vi "Wavelet Transform Daubechies4.vi"(0 "X":dbl[](array[numeric])) -> (1 "Wavelet Daubechies4 {X}":dbl[](array[numeric]), 2 "error":i32)   [LabVIEW 2010, in "NI_Gmath.lvlib"]
doc: "Computes the wavelet transform based on the Daubechies4 function of the input sequence <B>X</B>."
uses:
  NI_Gmath.lvlib
  Real Dot Product.vi
  NI_AALBase.lvlib
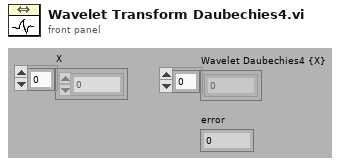
[diagram p1: front panel]
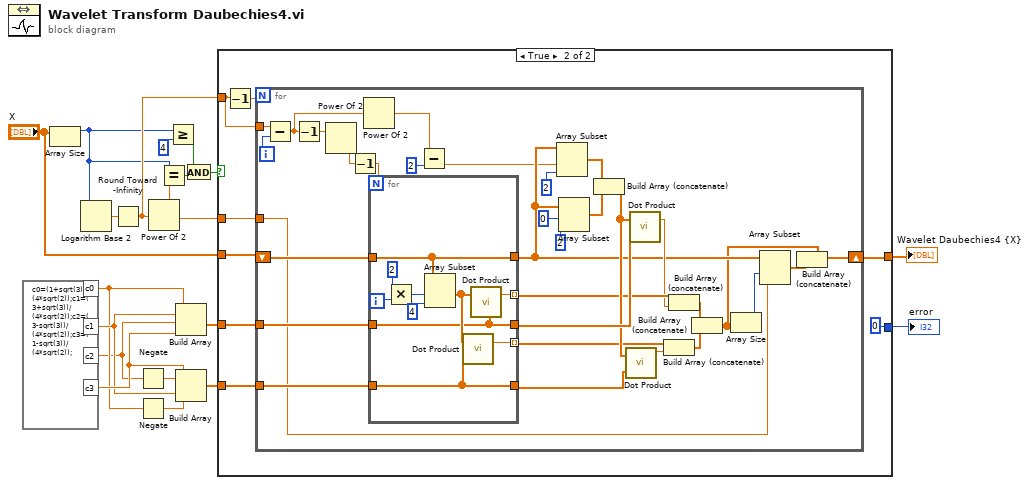
[diagram p0: block diagram]
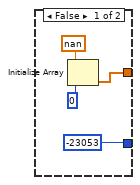
[diagram p2: hidden frame]
diagram:
  n1 = formula code="c0=(1+sqrt(3))/(4*sqrt(2));c1=(3+sqrt(3))/(4*sqrt(2));c2=(3-sqrt(3))/(4*sqrt(2));c3=(1-sqrt(3))/(4*sqrt(2));"() -> ("c0"=w7:dbl, "c1"=w10:dbl, "c2"=w6:dbl, "c3"=w11:dbl)
  n2 = Array Size(array="X") -> (size(s)=w2:i32)
  n3 = Logarithm Base 2(1:w2) -> (0:w19:dbl)
  n4 = Round Toward -Infinity(1:w19) -> (0:w12:dbl)
  n5 = Negate(x=w6) -> (-x=w9:dbl)
  n6 = Negate(x=w7) -> (-x=w8:dbl)
  n7 = Power Of 2(x=w12) -> (2^x=w18:dbl)
  n8 = Equal?(x=w2, y=w18) -> (x = y?=w14:bool)
  n9 = Greater Or Equal?(x=w2, y=4) -> (x >= y?=w15:bool)
  n10 = Build Array(w7, w10, w6, w11) -> (w4:dbl[])
  n11 = Build Array(w11, w9, w10, w8) -> (w5:dbl[])
  n12 = And(x=w15, y=w14) -> (x .and. y?=w13:bool)
  n13 = case shown="True" w13 {
    tunnel: [-23053 0] -> w17
    tunnel: w12 -> [_ w25]
    tunnel: "X" -> [_ w30]
    tunnel: w4 -> [_ w29]
    tunnel: w5 -> [_ w28]
    tunnel: w18 -> [_ w27]
    tunnel: [w20 w26] -> w1
    frame False {
      n14 = Initialize Array(nan, 0) -> (w20:dbl[])
    }
    frame True {
      n15 = Decrement(x=w25) -> (x-1=w24:dbl)
      n16 = for {
        N: w24 -> [_]
        tunnel: w25 -> [w37]
        shift-right: [w32] -> w26
        shift-left: w30 -> [w62]
        tunnel: w29 -> [w61]
        tunnel: w28 -> [w60]
        tunnel: w27 -> [w43]
        i -> [w63]
        n17 = Subtract(x=w37, y=w63) -> (x-y=w36:dbl)
        n18 = Decrement(x=w36) -> (x-1=w40:dbl)
        n19 = Power Of 2(x=w40) -> (2^x=w41:dbl)
        n20 = Decrement(x=w41) -> (x-1=w38:dbl)
        n21 = Power Of 2(x=w36) -> (2^x=w34:dbl)
        n22 = for {
          N: w38 -> [_]
          tunnel: w62 -> [w68]
          tunnel: w61 -> [w67]
          tunnel: w60 -> [w66]
          tunnel: [w68] -> w45
          tunnel: [w67] -> w54
          tunnel: [w66] -> w53
          tunnel: [w65] -> w51 mode=indexing
          tunnel: [w64] -> w49 mode=indexing
          i -> [w73]
          n23 = Multiply(x=2, y=w73) -> (x*y=w71:i32)
          n24 = Array Subset(array=w68, index=w71, length=4) -> (w69:dbl[])
          n25 = call-poly "Dot Product.vi"("Y Vector"=w66, "X Vector"=w69) -> ("X * Y"=w64:dbl)  [unwired: 1 out]
          n26 = call-poly "Dot Product.vi"("Y Vector"=w67, "X Vector"=w69) -> ("X * Y"=w65:dbl)  [unwired: 1 out]
        }
        n27 = Subtract(x=w34, y=2) -> (x-y=w33:dbl)
        n28 = Array Subset(array=w45, index=w33, length=2) -> (w56:dbl[])
        n29 = Array Subset(array=w45, index=0, length=2) -> (w55:dbl[])
        n30 = Build Array (concatenate)(w56, w55) -> (w52:dbl[])
        n31 = call-poly "Dot Product.vi"("Y Vector"=w53, "X Vector"=w52) -> ("X * Y"=w48:dbl)  [unwired: 1 out]
        n32 = call-poly "Dot Product.vi"("Y Vector"=w54, "X Vector"=w52) -> ("X * Y"=w50:dbl)  [unwired: 1 out]
        n33 = Build Array (concatenate)(w49, w48) -> (w46:dbl[])
        n34 = Build Array (concatenate)(w51, w50) -> (w47:dbl[])
        n35 = Build Array (concatenate)(w47, w46) -> (w39:dbl[])
        n36 = Array Size(array=w39) -> (size(s)=w44:i32)
        n37 = Array Subset(array=w45, index=w44, length=w43) -> (w42:dbl[])
        n38 = Build Array (concatenate)(w39, w42) -> (w32:dbl[])
      }
    }
  }
  "error" <- w17
  "Wavelet Daubechies4 {X}" <- w1
